vi "Relink Nodes.vi"(8 "error in (no error)":errorcluster, 10 "VI FQN":string, 11 "Path":path) -> (0 "error out":errorcluster)   [LabVIEW 2020, in "WebView2 Updater.lvclass"]
uses:
  WebView2 Updater.lvclass
  <vilib>/Utility/traverseref.llb/TRef TravTarget.ctl
  WebView2 Updater.lvclass/WebView2 Updater.ctl
  <vilib>/Utility/traverseref.llb/VI Scripting - Traverse.lvlib
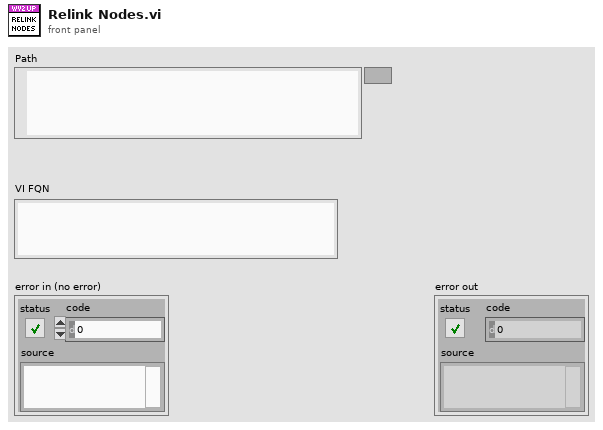
[diagram p1: front panel]
types:
  T1 = typedef "TRef TravTarget.ctl" = enum16{"FP", "BD", "Other"}
  T2 = typedef "ASPM_UniqueIDStringDatanameShortnameLongname.ctl" = cluster{"Unique ID string":string, "Data name":string, "Short name (localized)":string, "Long name (localized)":string}
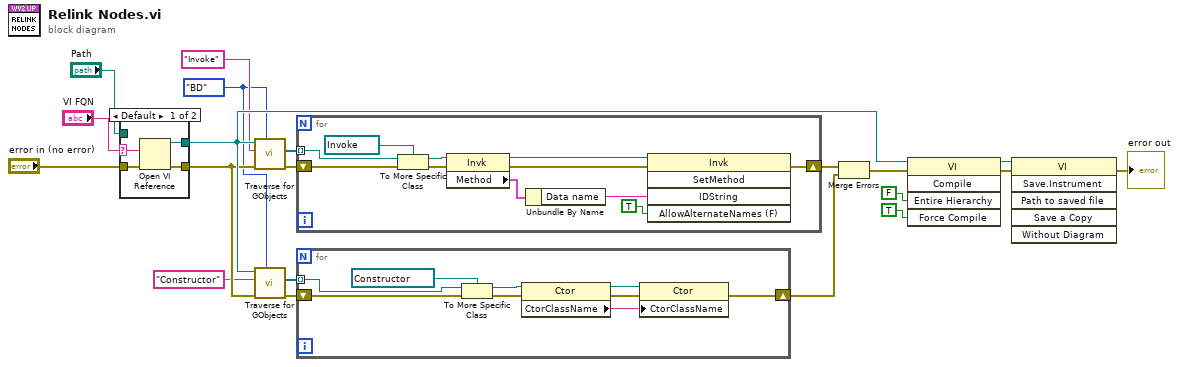
[diagram p0: block diagram]
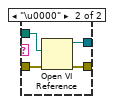
[diagram p2: hidden frame]
diagram:
  w10 = TRef_TravTarget."BD" ("Traverse Target")
  n1 = case shown="Default" "VI FQN" {
    selector: "VI FQN" -> [w22 _]
    tunnel: "Path" -> [_ w28]
    tunnel: [w21 w27] -> w19
    tunnel: "error in (no error)" -> [w24 w26]
    tunnel: [w23 w25] -> w14
    frame Default {
      n2 = Open VI Reference(vi path=w22, error in (no error)=w24) -> (vi reference=w21:refnum<vi>, error out=w23:errorcluster)  [unwired: 4 in]
    }
    frame "\u0000" {
      n3 = Open VI Reference(vi path=w28, error in (no error)=w26) -> (vi reference=w27:refnum<vi>, error out=w25:errorcluster)  [unwired: 4 in]
    }
  }
  n4 = call <vilib>:"Traverse for GObjects.vi"("Traverse Target"=w10, "error in (no error)"=w14, "Class Name"="Invoke", "VI Refnum"=w19) -> ("error out"=w13:errorcluster, "References"=w12:refnum<vi>[])  [unwired: 4 in, 2 out]
  n5 = call <vilib>:"Traverse for GObjects.vi"("Traverse Target"=w10, "error in (no error)"=w14, "Class Name"="Constructor", "VI Refnum"=w19) -> ("error out"=w9:errorcluster, "References"=w8:refnum<vi>[])  [unwired: 4 in, 2 out]
  n6 = for {
    tunnel: w12 -> [w39] mode=indexing
    shift-right: [w30] -> w15
    shift-left: w13 -> [w38]
    n7 = To More Specific Class(target class=refnum<vi> refnum ("References"), reference=w39, error in=w38) -> (specific class reference=w33:refnum<vi>, error out=w32:errorcluster)
    n8 = property class="Invk"(reference=w33, error in=w32) -> (reference out=w37:refnum<vi>, error out=w36:errorcluster, "Method"=w34:T2)
    n9 = Unbundle By Name(w34) -> ("Data name"=w35:string)
    n10 = invoke class="Invk" method="SetMethod"(reference=w37, error in=w36, "IDString"=w35, "AllowAlternateNames (F)"=TRUE ("Allow Alternate Names? (F)")) -> (error out=w30:errorcluster)  [unwired: 1 in, 4 out]
  }
  n11 = for {
    tunnel: w8 -> [w48] mode=indexing
    shift-right: [w43] -> w16
    shift-left: w9 -> [w47]
    n12 = To More Specific Class(target class=refnum<vi> refnum ("References"), reference=w48, error in=w47) -> (specific class reference=w41:refnum<vi>, error out=w46:errorcluster)
    n13 = property class="Ctor"(reference=w41, error in=w46) -> (reference out=w42:refnum<vi>, error out=w45:errorcluster, "CtorClassName"=w44:string)
    n14 = property class="Ctor"(reference=w42, error in=w45, "CtorClassName"=w44) -> (error out=w43:errorcluster)  [unwired: 1 out]
  }
  n15 = Merge Errors(w15, w16) -> (w2:errorcluster)
  n16 = invoke class="VI" method="Compile"(reference=w19, error in=w2, "Entire Hierarchy"=FALSE ("Compile Entire Hierarchy (F)"), "Force Compile"=TRUE ("Force Compile (T)")) -> (reference out=w3:refnum<vi>, error out=w6:errorcluster)  [unwired: 1 in, 3 out]
  n17 = invoke class="VI" method="Save.Instrument"(reference=w3, error in=w6) -> (error out=→"error out":errorcluster)  [unwired: 4 in, 5 out]
